vi "Play Evil Lough.vi"(8 "error in (no error)":errorcluster, 10 "Number of games":i32, 11 "Application in":refnum<class "Application.lvclass">) -> (0 "error out":errorcluster, 3 "Application out":refnum<class "Application.lvclass">)   [LabVIEW 2021, in "Application.lvclass"]
uses:
  Application.lvclass
  LVApp/Modules/Sound Manager/Typedefs/Sound Effects.ctl
  Application.lvclass/Application.ctl
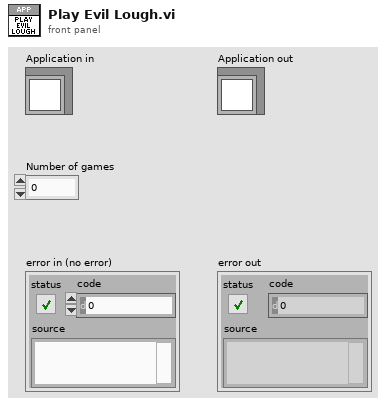
[diagram p1: front panel]
types:
  T1 = typedef "Sound Effects.ctl" = enum16{"Bomb In", "Bomb Out", "Bomb Touched", "Game Over", "Victory", "Eat", "10 Fruits", "Eat2", "Eat3", "Eat4", "MaxShield", "Shield", "10p", "Grape In", "Grape Out", "20p", "30p", "40p", "50p", "60p", "70p", "80p", "90p", "100p", "All shields cracked", "Mouse In", "Mouse Out", "Mouse Eaten", "Grape Eaten", "States Recover", "Broken Shield", "Bonus", "Happy Time", "explode", "Game over musica", "Back Music", "Shield Catch", "Evil lough", "Cricket In", "Cricket eaten", "Lets Go", "Jump1", "Jump2", "Jump3", "Unstoppable", "Troll Music", "winner"}
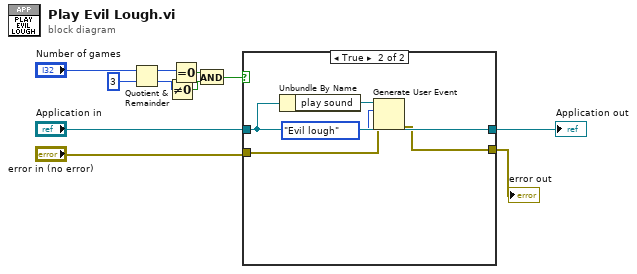
[diagram p0: block diagram]
diagram:
  n1 = Quotient & Remainder(x="Number of games", y=3) -> (x-y*floor(x/y)=w3:i32, floor(x/y)=w8:i32)
  n2 = Not Equal To 0?(x=w8) -> (x != 0?=w10:bool)
  n3 = Equal To 0?(x=w3) -> (x = 0?=w7:bool)
  n4 = And(x=w7, y=w10) -> (x .and. y?=w9:bool)
  n5 = case shown="True" w9 {
    tunnel: "Application in" -> [w13 w18]
    tunnel: [w13 w18] -> w5
    tunnel: "error in (no error)" -> [w12 w15]
    tunnel: [w12 w14] -> w11
    frame False {
    }
    frame True {
      n6 = Unbundle By Name(w18) -> ("play sound"=w17:refnum<user-event>)
      n7 = Generate User Event(user event=w17, event data cluster=Sound_Effects."Evil lough" ("event data"), error in=w15) -> (error out=w14:errorcluster)  [unwired: 1 in, 1 out]
    }
  }
  "error out" <- w11
  "Application out" <- w5
